vi "VI Tree.vi"   [LabVIEW 2016, in "Error Manager.lvlib" / "MHL Queue.lvclass"]
doc: "VI Tree\nThis VI lists all the public VIs and CTLs of the library."
uses:
  MHL Queue.lvclass
  Command (enum).ctl
panel:
  # "VI Tree\nSee the block diagram for the VI Tree"
types:
  T1 = typedef "Error Manager.lvlib/MHL Queue.lvclass/Command (enum).ctl" = enum16{"Init Module", "Close Module", "Internal Error", "Create Error Log File", "Show Front Panel", "Handle Error", "Refresh MCL", "MCL Value Change", "Change Display Order", "One-Second Interval Expired", "Mark Selected Errors As Read", "Mark All Errors As Read", "Refresh Button State - MSEAR", "Refresh Button State - MAEAR"}
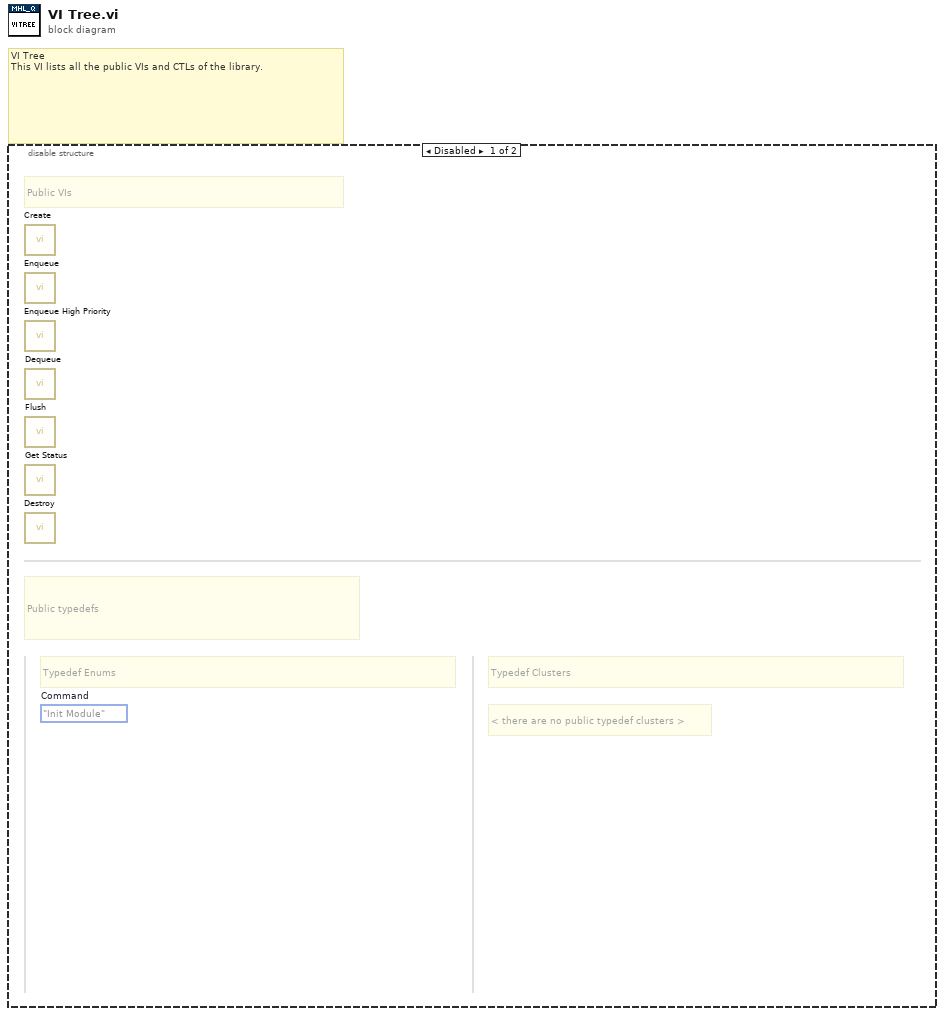
[diagram p0: block diagram]
diagram:
  # "VI Tree\nThis VI lists all the public VIs and CTLs of the library."
  n1 = disable-structure shown="Disabled" {
    frame Disabled {
      (unwired) Command_(enum)."Init Module"  # Command
      # "< there are no public typedef clusters >"
      # "Typedef Clusters"
      # "Typedef Enums"
      # "Public typedefs"
      # "Public VIs"
      n2 = call "Create.vi"() -> ()  [unwired: 11 in, 1 out]
      n3 = call "Enqueue.vi"() -> ()  [unwired: 11 in, 1 out]
      n4 = call "Enqueue High Priority.vi"() -> ()  [unwired: 11 in, 1 out]
      n5 = call "Dequeue.vi"() -> ()  [unwired: 9 in, 3 out]
      n6 = call "Flush.vi"() -> ()  [unwired: 9 in, 3 out]
      n7 = call "Get Status.vi"() -> ()  [unwired: 9 in, 3 out]
      n8 = call "Destroy.vi"() -> ()  [unwired: 9 in, 3 out]
    }
    frame Enabled {
    }
  }
